vi "AI color scada.vi"(8 "error in":errorcluster, 9 "change":bool, 10 "AIState":T1[](array[typedef]), 11 "AI_refs":refnum<vi>[](array[refnum])) -> (0 "error":errorcluster)   [LabVIEW 2019, in "Inputs.lvlib"]
uses:
  Inputs.lvlib
  Ctl/Parameter State.ctl
  Userlib.lvlib
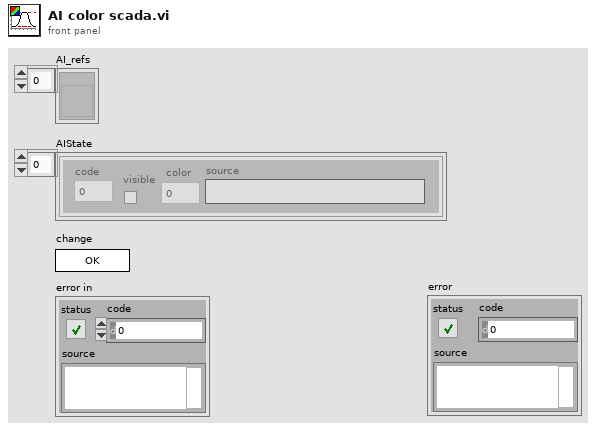
[diagram p1: front panel]
types:
  T1 = typedef "Inputs.lvlib/Parameter State.ctl" = cluster{"code":i32, "visible":bool, "color":u32, "source":string}
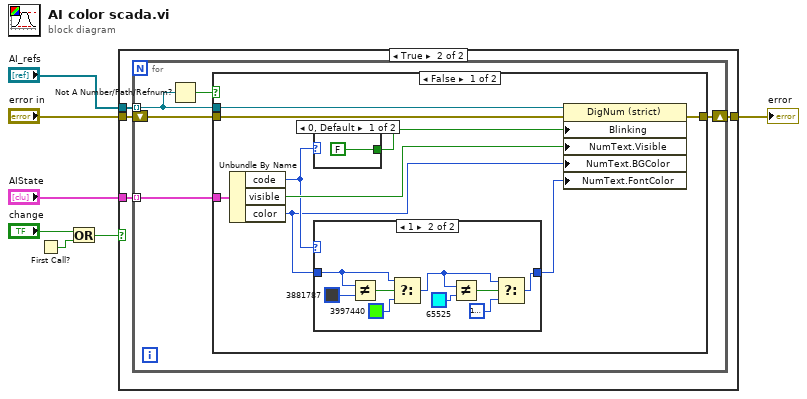
[diagram p0: block diagram]
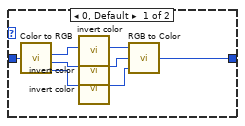
[diagram p3: hidden frame]
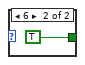
[diagram p4: hidden frame]
diagram:
  n1 = First Call?() -> (First Call?: T/F=w1:bool)
  n2 = Or(x="change", y=w1) -> (x .or. y?=w2:bool)
  n3 = case shown="True" w2 {
    tunnel: [w8 w12] -> w4
    tunnel: "error in" -> [w8 w11]
    tunnel: "AI_refs" -> [_ w10]
    tunnel: "AIState" -> [_ w9]
    frame False {
    }
    frame True {
      n4 = for {
        tunnel: w10 -> [w14] mode=indexing
        tunnel: w9 -> [w17] mode=indexing
        shift-right: [w15] -> w12
        shift-left: w11 -> [w16]
        n5 = Not A Number/Path/Refnum?(number/path/refnum=w14) -> (NaN/Path/Refnum?=w13:bool)
        n6 = case shown="False" w13 {
          tunnel: w17 -> [w26 _]
          tunnel: w16 -> [w25 w46]
          tunnel: [w24 w46] -> w15
          tunnel: w14 -> [w22 _]
          frame False {
            n7 = Unbundle By Name(w26) -> ("code"=w20:i32, "visible"=w21:bool, "color"=w19:u32)
            n8 = case shown="0, Default" w20 {
              tunnel: [FALSE TRUE] -> w23
              frame 0, Default {
              }
              frame 6 {
              }
            }
            n9 = case shown="1" w20 {
              tunnel: w19 -> [w28 w40]
              tunnel: [w27 w35] -> w18
              frame 0, Default {
                n10 = call <vilib>:"Color to RGB.vi"("Color"=w28) -> ("R"=w34:u8, "G"=w32:u8, "B"=w29:u8)  [unwired: 1 out]
                n11 = call "invert color.vi"("color"=w34) -> ("invert color"=w33:u8)  [unwired: 10 in]
                n12 = call "invert color.vi"("color"=w32) -> ("invert color"=w31:u8)  [unwired: 10 in]
                n13 = call "invert color.vi"("color"=w29) -> ("invert color"=w30:u8)  [unwired: 10 in]
                n14 = call <vilib>:"RGB to Color.vi"("B"=w30, "G"=w31, "R"=w33) -> ("Color"=w27:u32)
              }
              frame 1 {
                n15 = Not Equal?(x=w40, y=u32 3881787 ("color")) -> (x != y?=w43:bool)
                n16 = Select(t=w40, s=w43, f=u32 3997440 ("color")) -> (s? t:f=w37:u32)
                n17 = Not Equal?(x=w37, y=u32 65525 ("color")) -> (x != y?=w38:bool)
                n18 = Select(t=w37, s=w38, f=u32 16777222 ("color")) -> (s? t:f=w35:u32)
              }
            }
            n19 = property on="Property Node" class="DigNum (strict)"(reference=w22, error in=w25, "Blinking"=w23, "NumText.Visible"=w21, "NumText.BGColor"=w19, "NumText.FontColor"=w18) -> (error out=w24:errorcluster)  [unwired: 1 out]
          }
          frame True {
          }
        }
      }
    }
  }
  "error" <- w4
